vi "Wait for Server.vi"(8 "error in (no error)":errorcluster, 10 "loop delay (100ms)":dbl[unit]=0.1, 11 "Timeout (10s)":dbl[unit]=10000.0) -> (0 "error out":errorcluster)   [LabVIEW 2009, in "HighFinesse WS5.lvlib"]
doc: "Waits for a server to be active, and returns either when one is active or after timing out."
uses:
  HighFinesse WS5.lvlib
  <vilib>/Utility/error.llb/DialogType.ctl
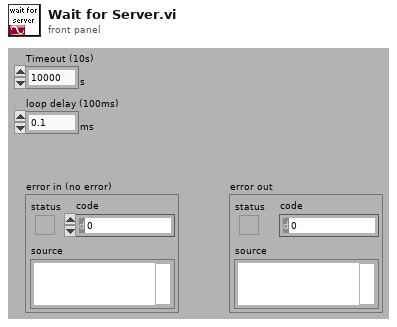
[diagram p1: front panel]
types:
  T1 = typedef "DialogType.ctl" = u16
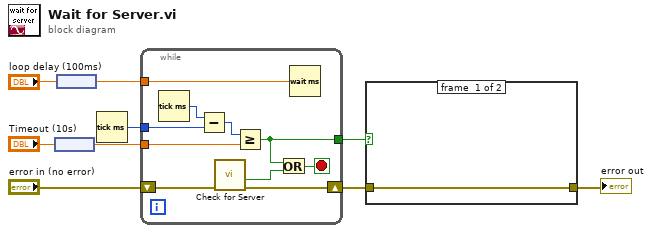
[diagram p0: block diagram]
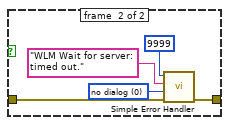
[diagram p2: hidden frame]
diagram:
  n1 = node("Timeout (10s)") -> (w1:dbl)
  n2 = node("loop delay (100ms)") -> (w3:dbl)
  n3 = Tick Count (ms)() -> (millisecond timer value=w8:u32)
  n4 = while {
    shift-right: [w19] -> w6
    shift-left: "error in (no error)" -> [w18]
    tunnel: w8 -> [w16]
    tunnel: w1 -> [w14]
    tunnel: [w11] -> w7
    tunnel: w3 -> [w10]
    stop <- w12 stop-if-true
    n5 = Tick Count (ms)() -> (millisecond timer value=w17:u32)
    n6 = Subtract(x=w17, y=w16) -> (x-y=w15:u32)
    n7 = call "Check for Server.vi"("error in (no error)"=w18) -> ("error out"=w19:errorcluster, "WLM server running?"=w13:bool)  [unwired: 9 out]
    n8 = Greater Or Equal?(x=w15, y=w14) -> (x >= y?=w11:bool)
    n9 = Or(x=w11, y=w13) -> (x .or. y?=w12:bool)
    n10 = Wait (ms)(milliseconds to wait=w10) -> ()  [unwired: 1 out]
  }
  n11 = case shown="True" w7 {
    tunnel: w6 -> [w20 w25]
    tunnel: [w20 w21] -> w5
    frame #0 {
    }
    frame #1 {
      w23 = T1 0 items=["no dialog", "OK message", "continue or stop message", "OK message + warnings", "continue/stop + warnings"] ("type of dialog (OK msg:1)")
      n12 = call <vilib>:"Simple Error Handler.vi"("error code (no error:0)"=9999, "error source (\" \")"="WLM Wait for server: timed out." ("error source (\" \")"), "type of dialog (OK msg:1)"=w23, "error in (no error)"=w25) -> ("error out"=w21:errorcluster)  [unwired: 5 out]
    }
  }
  "error out" <- w5
